vi "Simulated VeriStand Engine.Get Total Channel Count.vi"(8 "error in (no error)":errorcluster, 11 "Simulated VeriStand Engine in":refnum<class "Simulated VeriStand Engine.lvclass">) -> (0 "error out":errorcluster, 2 "total channel count":u32, 3 "Simulated VeriStand Engine out":refnum<class "Simulated VeriStand Engine.lvclass">)   [LabVIEW 2016, in "Simulated VeriStand Engine.lvclass"]
uses:
  Simulated VeriStand Engine.lvclass
  Simulated VeriStand Engine.lvclass/Simulated VeriStand Engine.ctl
  Simulated VeriStand Custom Device/Simulated VeriStand Custom Device.lvclass/Simulated VeriStand Custom Device.ctl
  Simulated VeriStand Custom Device/Simulated VeriStand Custom Device.lvclass
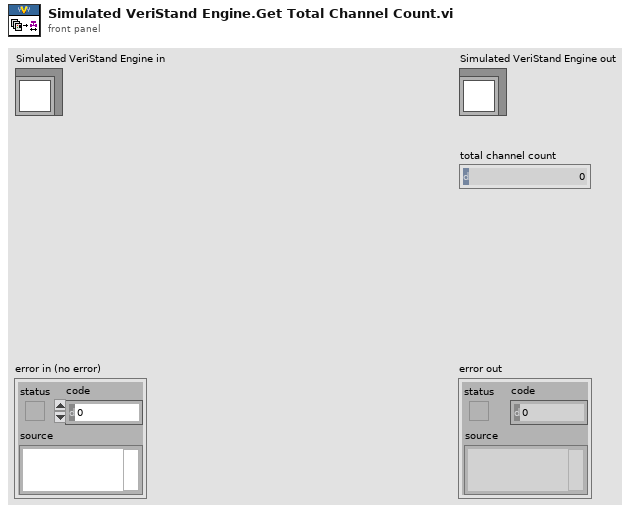
[diagram p1: front panel]
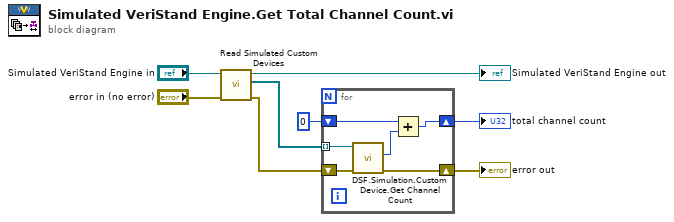
[diagram p0: block diagram]
diagram:
  n1 = call "Read Simulated Custom Devices.vi"("error in (no error)"="error in (no error)", "Simulated VeriStand Engine in"="Simulated VeriStand Engine in") -> ("error out"=w7:errorcluster, "Simulated Custom Devices"=w8:refnum<class "Simulated VeriStand Custom Device.lvclass">[], "Simulated VeriStand Engine out"=→"Simulated VeriStand Engine out":refnum<class "Simulated VeriStand Engine.lvclass">)  [unwired: 7 in]
  n2 = for {
    tunnel: w8 -> [w14] mode=indexing
    shift-right: [w12] -> w2
    shift-left: w7 -> [w13]
    shift-right: [w9] -> w1
    shift-left: u32 0 ("Channel Count") -> [w11]
    n3 = call "DSF.Simulation.Custom Device.Get Channel Count.vi"("error in (no error)"=w13, "Simulated VeriStand Custom Device in"=w14) -> ("error out"=w12:errorcluster, "Channel Count"=w10:u32)  [unwired: 7 in, 1 out]
    n4 = Add(x=w11, y=w10) -> (x+y=w9:u32)
  }
  "error out" <- w2
  "total channel count" <- w1
